vi "pump rpm.vi"(0 "flow rate":dbl[unit] format="%.2f", 1 "tubing size":enum16{"13", "14", "16", "25", "17", "18"}(ring)) -> (2 "pump speed":dbl[unit] format="%.2f", 3 "pump speed (rpm)":dbl format="%.2f", 4 "tube diameter":dbl[unit] format="%.2f", 5 "in range":bool)   [LabVIEW 2012]
uses:
  Pump calibration/calibration commands.ctl
panel:
  in  "diameter":dbl[unit][](array[numeric])=[0.00079375, 0.0015875, 0.003175, 0.004762499999999999, 0.00635, 0.0079375] format="%.5f"
  in  "pumpflow":dbl[unit][](array[numeric])=[9.549296547316535e-09, 3.342253804929783e-08, 1.2732395447351617e-07, 2.705634032562094e-07, 4.4563384065730255e-07, 6.04788783748884e-07] format="%.3f"
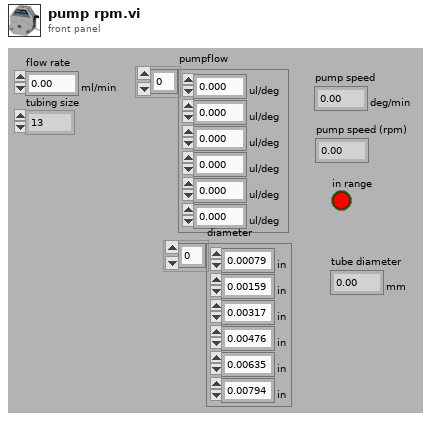
[diagram p1: front panel]
types:
  T1 = typedef "calibration commands.ctl" = enum16{"Get ini Path", "Save default values", "Save new calibration", "Read calibration", "Apply calibration", "Read STAMP mb", "Write STAMP mb"}
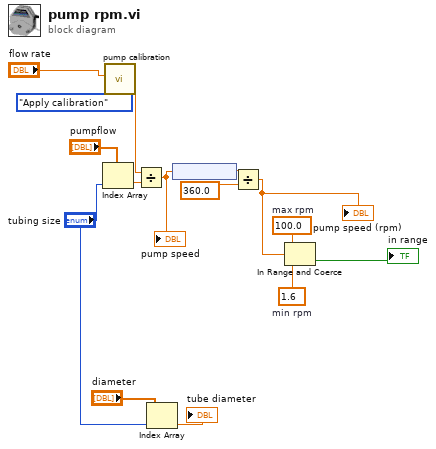
[diagram p0: block diagram]
diagram:
  w7 = 1.6  # min rpm
  w8 = 100.0  # max rpm
  n1 = Index Array(array="pumpflow", index="tubing size") -> (element=w14:dbl[unit])
  n2 = call "pump calibration.vi"("pump cal command"=calibration_commands."Apply calibration", "flow rate"="flow rate") -> ("modified flow rate"=w1:dbl[unit])  [unwired: 3 in, 3 out]
  n3 = Divide(x=w1, y=w14) -> (x/y=w13:dbl[unit])
  "pump speed" <- w13
  n4 = Index Array(array="diameter", index="tubing size") -> (element=→"tube diameter":dbl[unit])
  n5 = node(w13) -> (w12:dbl)
  n6 = Divide(x=w12, y=360.0) -> (x/y=w4:dbl)
  "pump speed (rpm)" <- w4
  n7 = In Range and Coerce(upper limit=w8, x=w4, lower limit=w7) -> (In Range?=→"in range":bool)  [unwired: 1 out]
